vi "0037-Sub_measure4.vi"(6 "数値":dbl, 7 "温湿度データ":dbl[][](array[numeric]), 8 "error out":errorcluster, 11 "device":T1) -> (0 "error out 2":errorcluster caption="error out", 2 "出力配列":dbl[](array[numeric]), 3 "device 2":T1, 4 "配列":bool[](array[boolean]), 5 "温湿度データ 2":dbl[][](array[numeric]))   [LabVIEW 2014]
uses:
  <userlib>/LV-CP2112_2014/LVProject/private/CP2112_device.ctl
  <userlib>/LV-CP2112_2014/LVProject/private/CP2112_SMBUS_S0.ctl
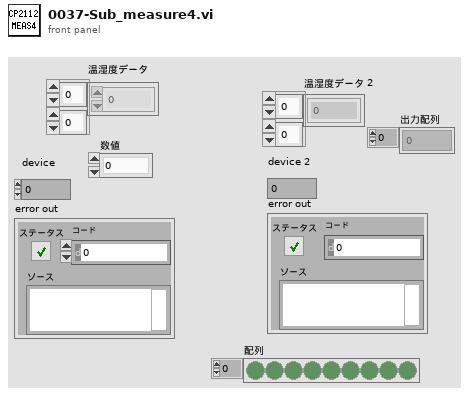
[diagram p1: front panel]
types:
  T1 = typedef "CP2112_device.ctl" = i32
  T2 = typedef "CP2112_SMBUS_S0.ctl" = enum8{"HID_SMBUS_S0_IDLE", "HID_SMBUS_S0_BUSY", "HID_SMBUS_S0_COMPLETE", "HID_SMBUS_S0_ERROR"}
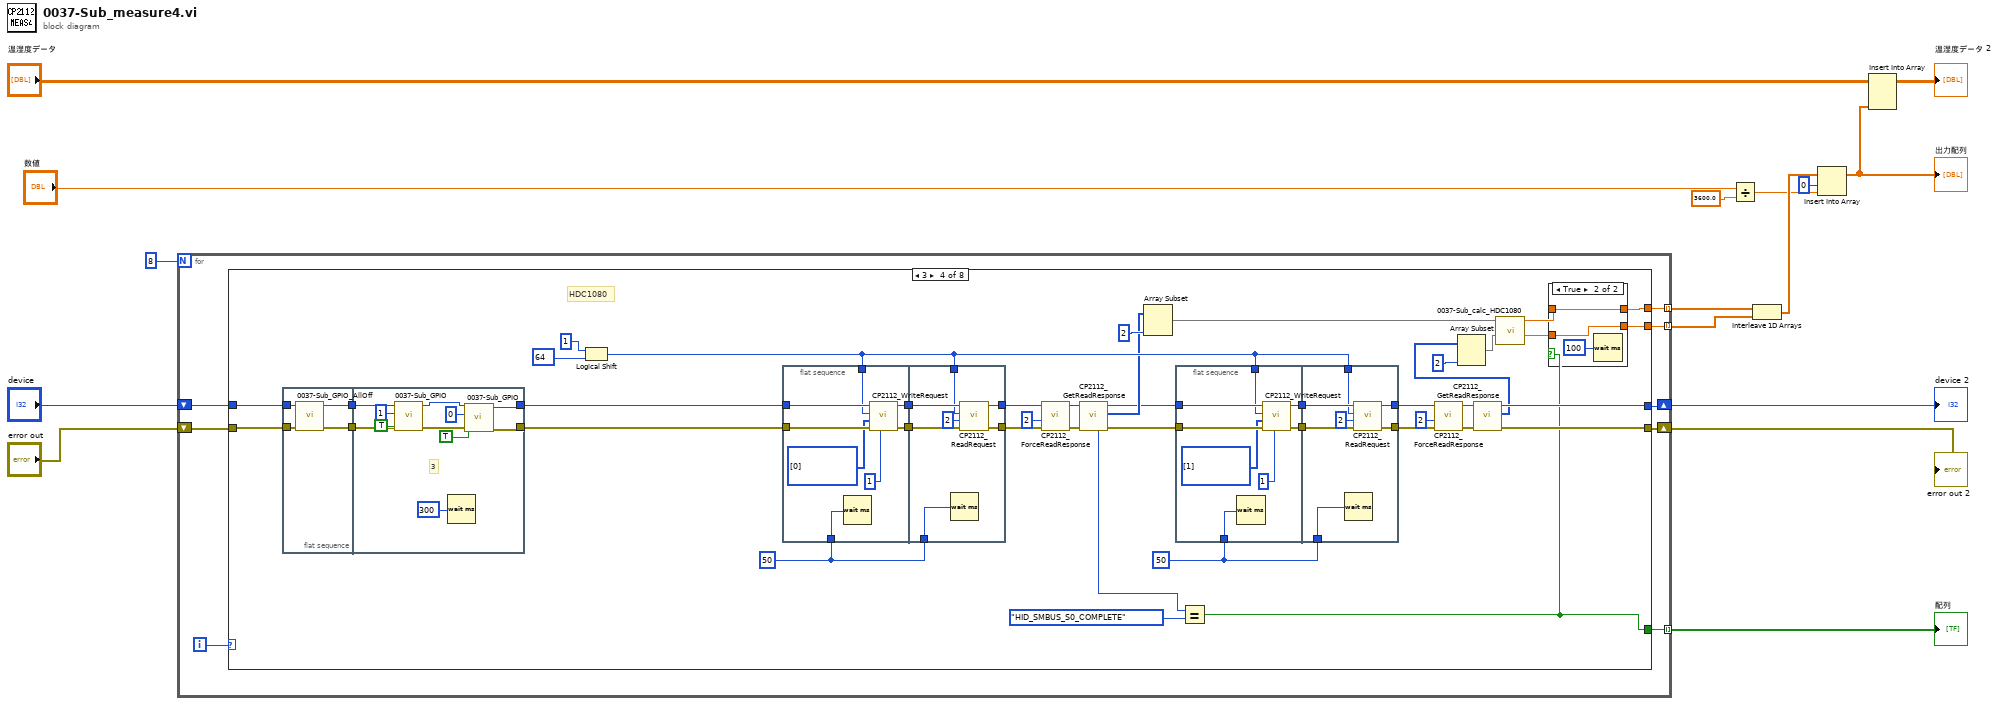
[diagram p0: block diagram]
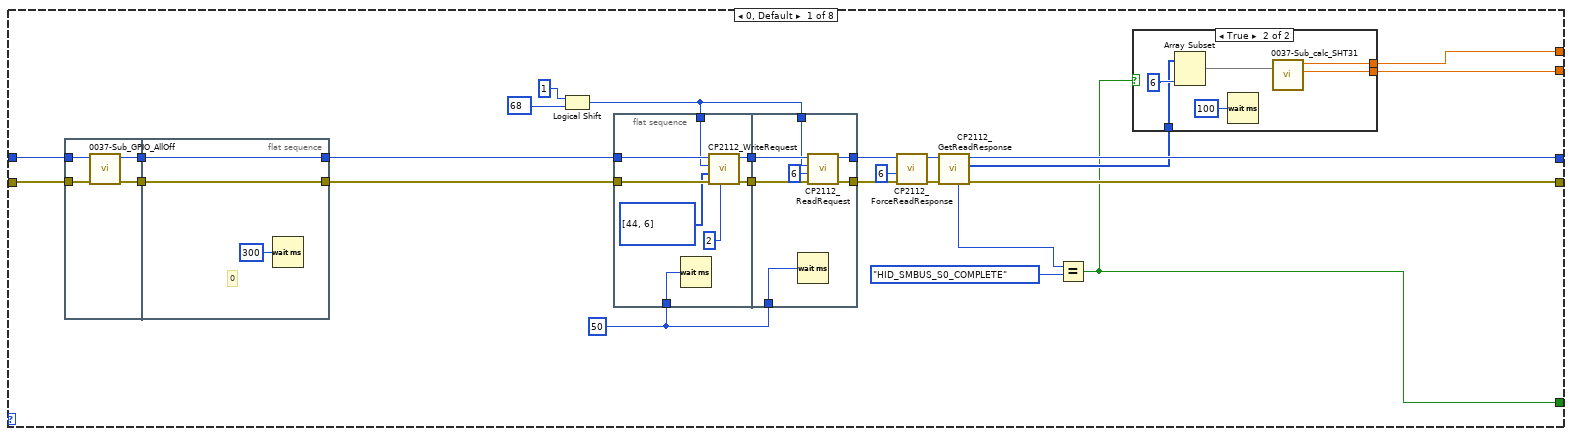
[diagram p2: hidden frame]
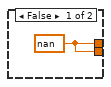
[diagram p3: hidden frame]
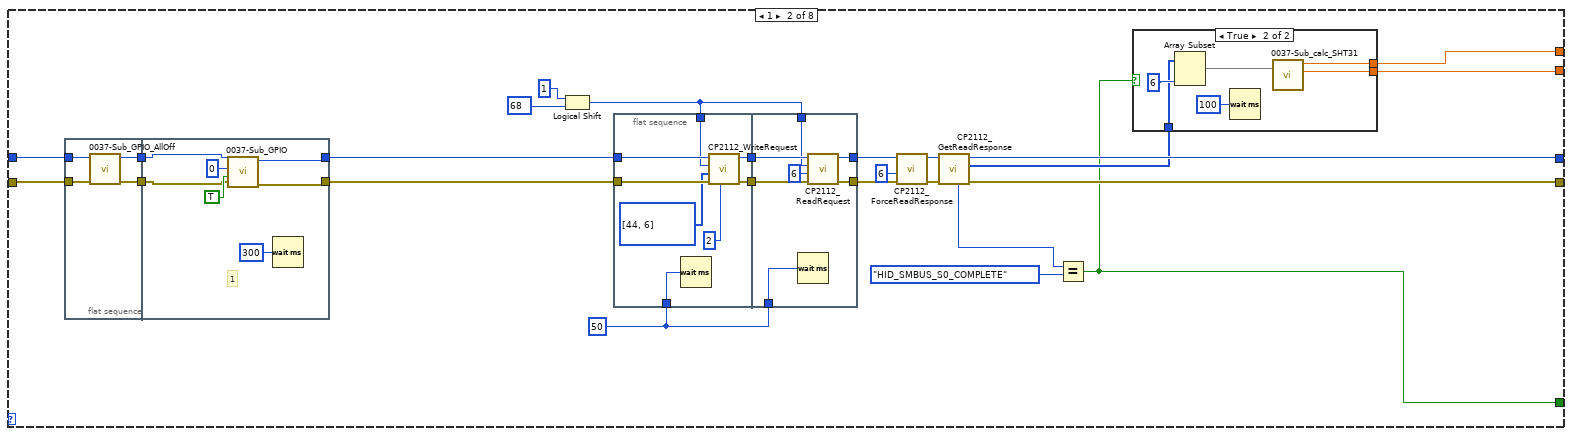
[diagram p4: hidden frame]
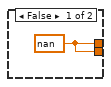
[diagram p5: hidden frame]
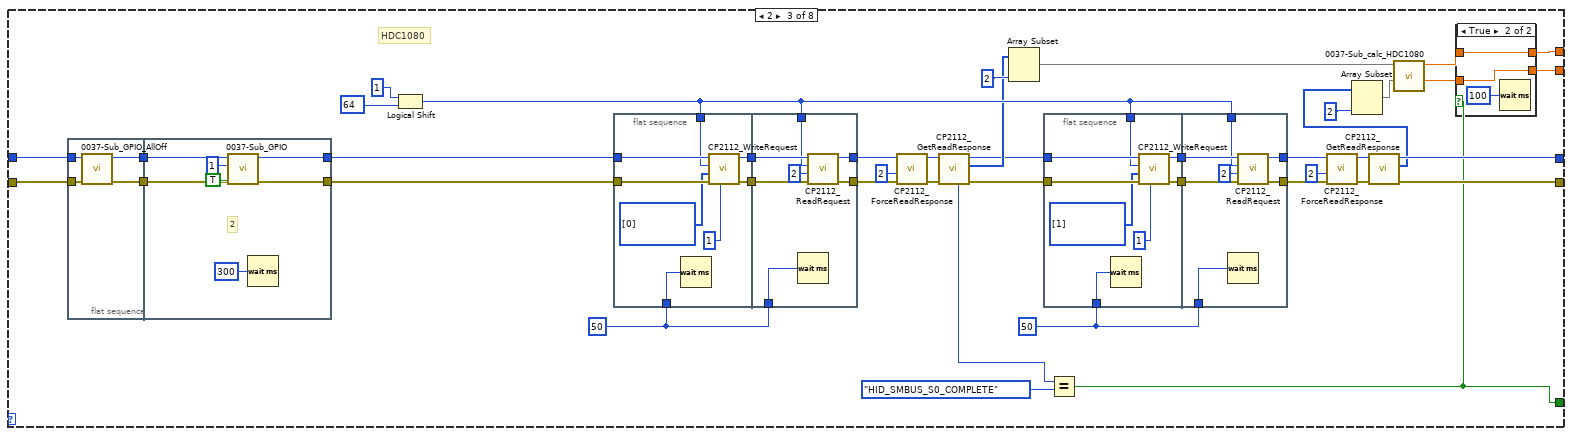
[diagram p6: hidden frame]
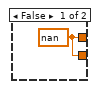
[diagram p7: hidden frame]
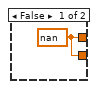
[diagram p8: hidden frame]
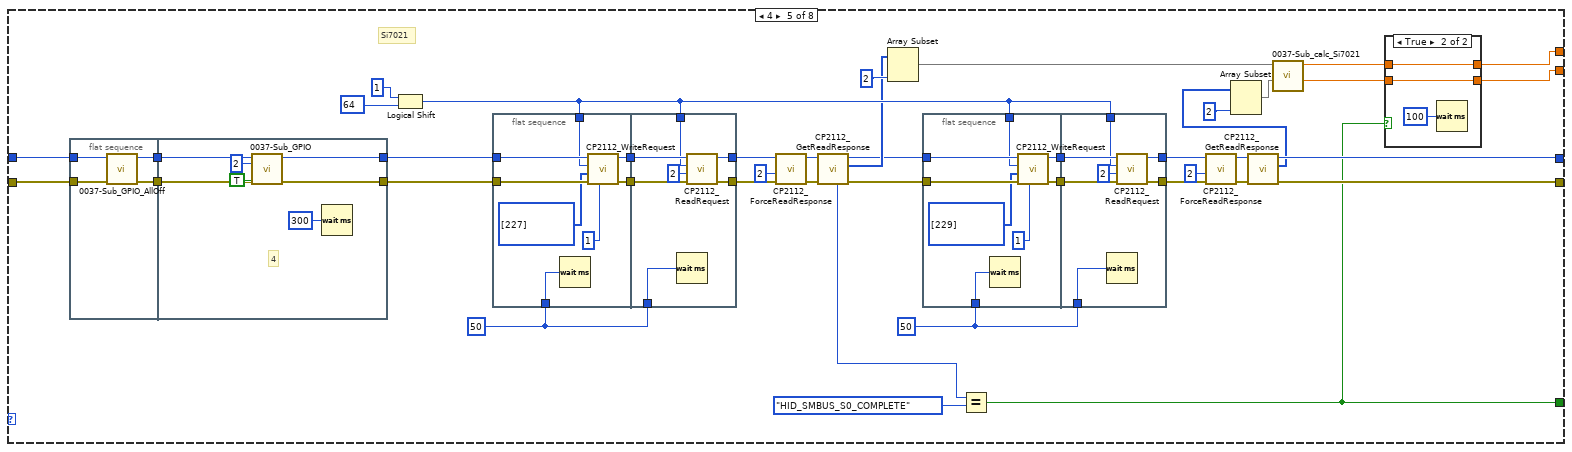
[diagram p9: hidden frame]
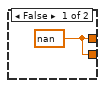
[diagram p10: hidden frame]
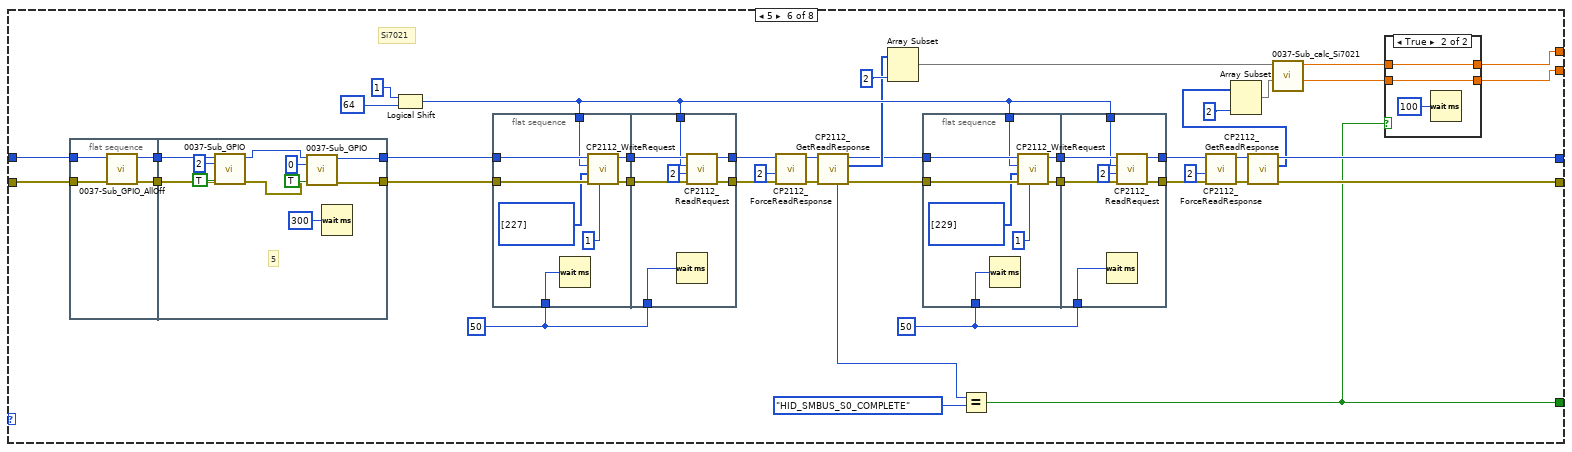
[diagram p11: hidden frame]
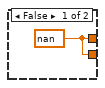
[diagram p12: hidden frame]
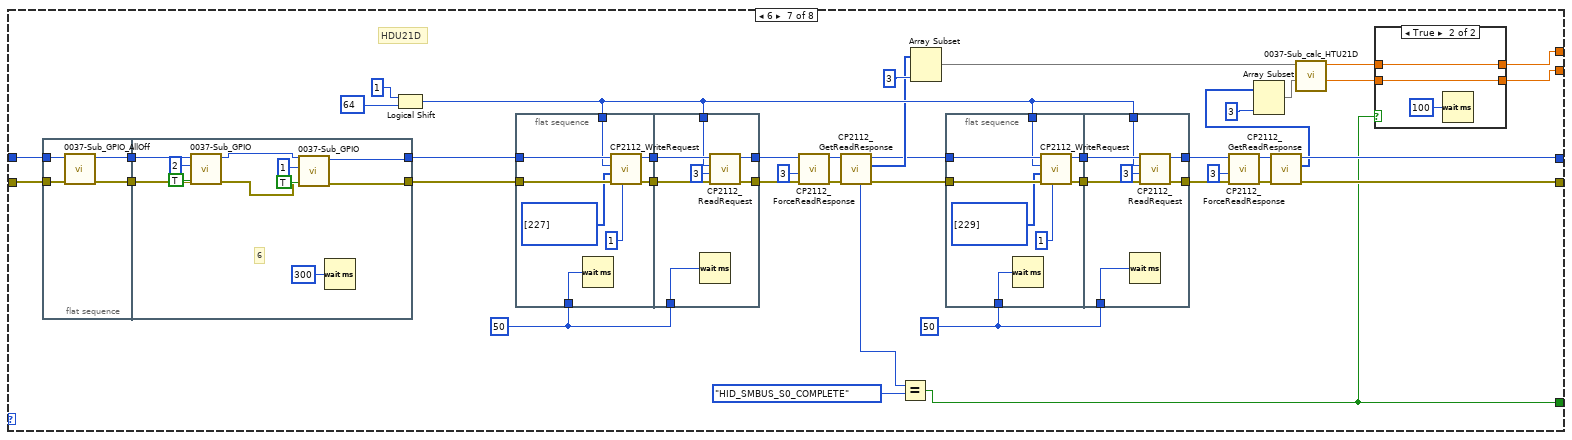
[diagram p13: hidden frame]
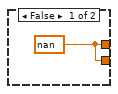
[diagram p14: hidden frame]
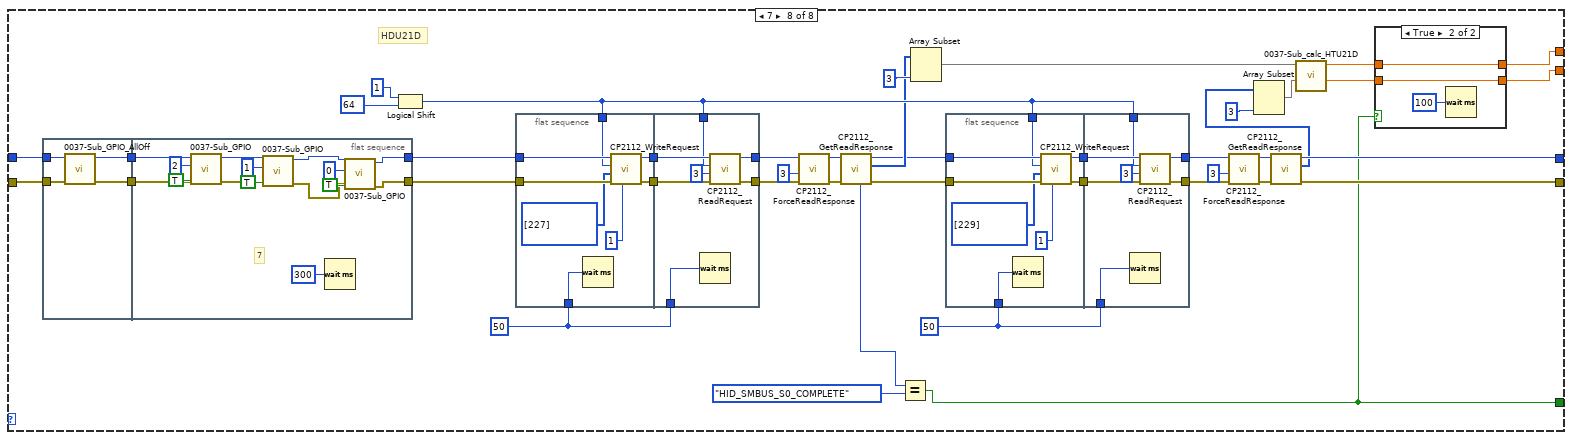
[diagram p15: hidden frame]
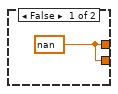
[diagram p16: hidden frame]
diagram:
  n1 = for {
    N: 8 -> [_]
    shift-right: [w22] -> w15
    shift-left: "error out" -> [w19]
    shift-right: [w23] -> w16
    shift-left: "device" -> [w18]
    tunnel: [w24] -> w14 mode=indexing
    tunnel: [w21] -> w9 mode=indexing
    tunnel: [w20] -> w8 mode=indexing
    i -> [w17]
    n2 = case shown="3" w17 {
      tunnel: [w25 w79 w137 w224 w319 w406 w497 w588] -> w24
      tunnel: [w41 w95 w172 w259 w350 w437 w528 w619] -> w23
      tunnel: [w42 w96 w173 w260 w351 w438 w529 w620] -> w22
      tunnel: [w44 w98 w139 w226 w318 w405 w496 w587] -> w21
      tunnel: [w43 w97 w141 w228 w316 w403 w494 w585] -> w20
      tunnel: w19 -> [w49 w103 w178 w265 w356 w443 w534 w625]
      tunnel: w18 -> [w48 w102 w177 w264 w355 w442 w533 w624]
      frame 0, Default {
        w30 = u32 50 ("ミリ秒待機時間")
        n3 = flat-sequence {
          tunnel: [w74] -> w40
          tunnel: [w72] -> w39
          tunnel: w48 -> [w75]
          tunnel: w49 -> [w73]
          tunnel: [w77] -> w27
          tunnel: [w78] -> w26
          tunnel: w40 -> [w77]
          tunnel: w39 -> [w78]
          frame #0 {
            n4 = call "0037-Sub_GPIO_AllOff.vi"("エラー出力 2"=w73, "device"=w75) -> ("エラー出力"=w72:errorcluster, "deviceOut"=w74:T1)  [unwired: 8 in]
          }
          frame #1 {
            # "0"
            n5 = Wait (ms)(milliseconds to wait=u32 300 ("ミリ秒待機時間")) -> ()  [unwired: 1 out]
          }
        }
        n6 = Logical Shift(y=1, x=68) -> (x << y=w45:i32)
        n7 = flat-sequence {
          tunnel: w26 -> [w64]
          tunnel: w27 -> [w63]
          tunnel: w45 -> [w58]
          tunnel: [w62] -> w38
          tunnel: [w61] -> w37
          tunnel: w30 -> [w57]
          tunnel: w38 -> [w69]
          tunnel: w37 -> [w68]
          tunnel: [w70] -> w32
          tunnel: [w67] -> w31
          tunnel: w45 -> [w66]
          tunnel: w30 -> [w65]
          frame #0 {
            n8 = Wait (ms)(milliseconds to wait=w57) -> ()  [unwired: 1 out]
            n9 = call <userlib>:"CP2112_WriteRequest.vi"("numBytesToWrite"=i16 2 ("numByteToRead"), "error in (no error)"=w64, "buffer"=u8[] [44, 6], "slaveAddress"=w58, "device"=w63) -> ("error out"=w62:errorcluster, "deviceOut"=w61:T1)  [unwired: 4 in, 1 out]
          }
          frame #1 {
            n10 = Wait (ms)(milliseconds to wait=w65) -> ()  [unwired: 1 out]
            n11 = call <userlib>:"CP2112_ReadRequest.vi"("error in (no error)"=w69, "numByteToRead"=i16 6, "slaveAddress"=w66, "device"=w68) -> ("error out"=w70:errorcluster, "deviceOut"=w67:T1)  [unwired: 5 in, 1 out]
          }
        }
        n12 = call <userlib>:"CP2112_ForceReadResponse.vi"("error in (no error)"=w32, "numByteToRead"=i16 6, "device"=w31) -> ("error out"=w36:errorcluster, "deviceOut"=w35:T1)  [unwired: 6 in, 1 out]
        n13 = call <userlib>:"CP2112_GetReadResponse.vi"("error in (no error)"=w36, "device"=w35) -> ("error out"=w42:errorcluster, "buffer"=w34:u8[], "deviceOut"=w41:T1, "HID_SMBUS_S0"=w29:T2)  [unwired: 4 in, 2 out]
        n14 = Equal?(x=w29, y=CP2112_SMBUS_S0."HID_SMBUS_S0_COMPLETE" ("HID_SMBUS_S0")) -> (x = y?=w25:bool)
        n15 = case shown="TRUE" w25 {
          tunnel: [w50 w56] -> w44
          tunnel: [w50 w55] -> w43
          tunnel: w34 -> [_ w52]
          frame False {
            w50 = nan ("数値 2")
          }
          frame True {
            n16 = Array Subset(array=w52, length=6 ("長さ")) -> (w54:u8[])  [unwired: 1 in]
            n17 = Wait (ms)(milliseconds to wait=u32 100 ("ミリ秒待機時間")) -> ()  [unwired: 1 out]
            n18 = call "0037-Sub_calc_SHT31.vi"("Data"=w54) -> ("数値"=w55:dbl, "数値 2"=w56:dbl)  [unwired: 9 in]
          }
        }
      }
      frame 1 {
        w84 = u32 50 ("ミリ秒待機時間")
        n19 = flat-sequence {
          tunnel: [w128] -> w94
          tunnel: [w126] -> w93
          tunnel: w102 -> [w129]
          tunnel: w103 -> [w127]
          tunnel: [w133] -> w81
          tunnel: [w132] -> w80
          tunnel: w94 -> [w130]
          tunnel: w93 -> [w131]
          frame #0 {
            n20 = call "0037-Sub_GPIO_AllOff.vi"("エラー出力 2"=w127, "device"=w129) -> ("エラー出力"=w126:errorcluster, "deviceOut"=w128:T1)  [unwired: 8 in]
          }
          frame #1 {
            # "1"
            n21 = call "0037-Sub_GPIO.vi"("エラー出力 2"=w131, "ブール"=TRUE, "GPIO"=u8 0, "device"=w130) -> ("エラー出力"=w132:errorcluster, "deviceOut"=w133:T1)  [unwired: 6 in]
            n22 = Wait (ms)(milliseconds to wait=u32 300 ("ミリ秒待機時間")) -> ()  [unwired: 1 out]
          }
        }
        n23 = Logical Shift(y=1, x=68) -> (x << y=w99:i32)
        n24 = flat-sequence {
          tunnel: w80 -> [w118]
          tunnel: w81 -> [w117]
          tunnel: w99 -> [w112]
          tunnel: [w116] -> w92
          tunnel: [w115] -> w91
          tunnel: w84 -> [w111]
          tunnel: w92 -> [w123]
          tunnel: w91 -> [w122]
          tunnel: [w124] -> w86
          tunnel: [w121] -> w85
          tunnel: w99 -> [w120]
          tunnel: w84 -> [w119]
          frame #0 {
            n25 = Wait (ms)(milliseconds to wait=w111) -> ()  [unwired: 1 out]
            n26 = call <userlib>:"CP2112_WriteRequest.vi"("numBytesToWrite"=i16 2 ("numByteToRead"), "error in (no error)"=w118, "buffer"=u8[] [44, 6], "slaveAddress"=w112, "device"=w117) -> ("error out"=w116:errorcluster, "deviceOut"=w115:T1)  [unwired: 4 in, 1 out]
          }
          frame #1 {
            n27 = Wait (ms)(milliseconds to wait=w119) -> ()  [unwired: 1 out]
            n28 = call <userlib>:"CP2112_ReadRequest.vi"("error in (no error)"=w123, "numByteToRead"=i16 6, "slaveAddress"=w120, "device"=w122) -> ("error out"=w124:errorcluster, "deviceOut"=w121:T1)  [unwired: 5 in, 1 out]
          }
        }
        n29 = call <userlib>:"CP2112_ForceReadResponse.vi"("error in (no error)"=w86, "numByteToRead"=i16 6, "device"=w85) -> ("error out"=w90:errorcluster, "deviceOut"=w89:T1)  [unwired: 6 in, 1 out]
        n30 = call <userlib>:"CP2112_GetReadResponse.vi"("error in (no error)"=w90, "device"=w89) -> ("error out"=w96:errorcluster, "buffer"=w88:u8[], "deviceOut"=w95:T1, "HID_SMBUS_S0"=w83:T2)  [unwired: 4 in, 2 out]
        n31 = Equal?(x=w83, y=CP2112_SMBUS_S0."HID_SMBUS_S0_COMPLETE" ("HID_SMBUS_S0")) -> (x = y?=w79:bool)
        n32 = case shown="TRUE" w79 {
          tunnel: [w104 w110] -> w98
          tunnel: [w104 w109] -> w97
          tunnel: w88 -> [_ w106]
          frame False {
            w104 = nan ("数値 2")
          }
          frame True {
            n33 = Array Subset(array=w106, length=6 ("長さ")) -> (w108:u8[])  [unwired: 1 in]
            n34 = Wait (ms)(milliseconds to wait=u32 100 ("ミリ秒待機時間")) -> ()  [unwired: 1 out]
            n35 = call "0037-Sub_calc_SHT31.vi"("Data"=w108) -> ("数値"=w109:dbl, "数値 2"=w110:dbl)  [unwired: 9 in]
          }
        }
      }
      frame 2 {
        w151 = u32 50 ("ミリ秒待機時間")
        w158 = u32 50 ("ミリ秒待機時間")
        # "HDC1080"
        n36 = flat-sequence {
          tunnel: [w215] -> w171
          tunnel: [w213] -> w170
          tunnel: w177 -> [w216]
          tunnel: w178 -> [w214]
          tunnel: [w223] -> w144
          tunnel: [w222] -> w145
          tunnel: w171 -> [w220]
          tunnel: w170 -> [w219]
          frame #0 {
            n37 = call "0037-Sub_GPIO_AllOff.vi"("エラー出力 2"=w214, "device"=w216) -> ("エラー出力"=w213:errorcluster, "deviceOut"=w215:T1)  [unwired: 8 in]
          }
          frame #1 {
            # "2"
            n38 = call "0037-Sub_GPIO.vi"("エラー出力 2"=w219, "ブール"=TRUE, "GPIO"=u8 1, "device"=w220) -> ("エラー出力"=w222:errorcluster, "deviceOut"=w223:T1)  [unwired: 6 in]
            n39 = Wait (ms)(milliseconds to wait=u32 300 ("ミリ秒待機時間")) -> ()  [unwired: 1 out]
          }
        }
        n40 = Logical Shift(y=1, x=64) -> (x << y=w174:i32)
        n41 = flat-sequence {
          tunnel: w145 -> [w205]
          tunnel: w144 -> [w204]
          tunnel: w174 -> [w199]
          tunnel: [w203] -> w169
          tunnel: [w202] -> w168
          tunnel: w158 -> [w198]
          tunnel: w169 -> [w210]
          tunnel: w168 -> [w209]
          tunnel: [w211] -> w160
          tunnel: [w208] -> w159
          tunnel: w174 -> [w207]
          tunnel: w158 -> [w206]
          frame #0 {
            n42 = Wait (ms)(milliseconds to wait=w198) -> ()  [unwired: 1 out]
            n43 = call <userlib>:"CP2112_WriteRequest.vi"("numBytesToWrite"=i16 1 ("numByteToRead"), "error in (no error)"=w205, "buffer"=u8[] [0], "slaveAddress"=w199, "device"=w204) -> ("error out"=w203:errorcluster, "deviceOut"=w202:T1)  [unwired: 4 in, 1 out]
          }
          frame #1 {
            n44 = Wait (ms)(milliseconds to wait=w206) -> ()  [unwired: 1 out]
            n45 = call <userlib>:"CP2112_ReadRequest.vi"("error in (no error)"=w210, "numByteToRead"=i16 2, "slaveAddress"=w207, "device"=w209) -> ("error out"=w211:errorcluster, "deviceOut"=w208:T1)  [unwired: 5 in, 1 out]
          }
        }
        n46 = call <userlib>:"CP2112_ForceReadResponse.vi"("error in (no error)"=w160, "numByteToRead"=i16 2, "device"=w159) -> ("error out"=w165:errorcluster, "deviceOut"=w164:T1)  [unwired: 6 in, 1 out]
        n47 = call <userlib>:"CP2112_GetReadResponse.vi"("error in (no error)"=w165, "device"=w164) -> ("error out"=w150:errorcluster, "buffer"=w162:u8[], "deviceOut"=w149:T1, "HID_SMBUS_S0"=w142:T2)  [unwired: 4 in, 2 out]
        n48 = Array Subset(array=w162, length=2 ("長さ")) -> (w157:u8[])  [unwired: 1 in]
        n49 = flat-sequence {
          tunnel: w150 -> [w190]
          tunnel: w149 -> [w189]
          tunnel: w174 -> [w184]
          tunnel: [w188] -> w167
          tunnel: [w187] -> w166
          tunnel: w151 -> [w183]
          tunnel: w167 -> [w195]
          tunnel: w166 -> [w194]
          tunnel: [w196] -> w153
          tunnel: [w193] -> w152
          tunnel: w174 -> [w192]
          tunnel: w151 -> [w191]
          frame #0 {
            n50 = Wait (ms)(milliseconds to wait=w183) -> ()  [unwired: 1 out]
            n51 = call <userlib>:"CP2112_WriteRequest.vi"("numBytesToWrite"=i16 1 ("numByteToRead"), "error in (no error)"=w190, "buffer"=u8[] [1], "slaveAddress"=w184, "device"=w189) -> ("error out"=w188:errorcluster, "deviceOut"=w187:T1)  [unwired: 4 in, 1 out]
          }
          frame #1 {
            n52 = Wait (ms)(milliseconds to wait=w191) -> ()  [unwired: 1 out]
            n53 = call <userlib>:"CP2112_ReadRequest.vi"("error in (no error)"=w195, "numByteToRead"=i16 2, "slaveAddress"=w192, "device"=w194) -> ("error out"=w196:errorcluster, "deviceOut"=w193:T1)  [unwired: 5 in, 1 out]
          }
        }
        n54 = Equal?(x=w142, y=CP2112_SMBUS_S0."HID_SMBUS_S0_COMPLETE" ("HID_SMBUS_S0")) -> (x = y?=w137:bool)
        n55 = call <userlib>:"CP2112_ForceReadResponse.vi"("error in (no error)"=w153, "numByteToRead"=i16 2, "device"=w152) -> ("error out"=w156:errorcluster, "deviceOut"=w155:T1)  [unwired: 6 in, 1 out]
        n56 = call <userlib>:"CP2112_GetReadResponse.vi"("error in (no error)"=w156, "device"=w155) -> ("error out"=w173:errorcluster, "buffer"=w146:u8[], "deviceOut"=w172:T1)  [unwired: 4 in, 3 out]
        n57 = Array Subset(array=w146, length=2 ("長さ")) -> (w147:u8[])  [unwired: 1 in]
        n58 = call "0037-Sub_calc_HDC1080.vi"("humi"=w147, "temp"=w157) -> ("humi"=w140:dbl, "temp"=w138:dbl)  [unwired: 7 in]
        n59 = case shown="TRUE" w137 {
          tunnel: [w179 w182] -> w141
          tunnel: w140 -> [_ w182]
          tunnel: [w179 w181] -> w139
          tunnel: w138 -> [_ w181]
          frame False {
            w179 = nan ("temp")
          }
          frame True {
            n60 = Wait (ms)(milliseconds to wait=u32 100 ("ミリ秒待機時間")) -> ()  [unwired: 1 out]
          }
        }
      }
      frame 3 {
        w238 = u32 50 ("ミリ秒待機時間")
        w245 = u32 50 ("ミリ秒待機時間")
        # "HDC1080"
        n61 = flat-sequence {
          tunnel: [w302] -> w258
          tunnel: [w300] -> w257
          tunnel: w264 -> [w303]
          tunnel: w265 -> [w301]
          tunnel: [w307] -> w231
          tunnel: [w306] -> w232
          tunnel: w258 -> [w313]
          tunnel: w257 -> [w312]
          frame #0 {
            n62 = call "0037-Sub_GPIO_AllOff.vi"("エラー出力 2"=w301, "device"=w303) -> ("エラー出力"=w300:errorcluster, "deviceOut"=w302:T1)  [unwired: 8 in]
          }
          frame #1 {
            # "3"
            n63 = call "0037-Sub_GPIO.vi"("エラー出力 2"=w312, "ブール"=TRUE, "GPIO"=u8 1, "device"=w313) -> ("エラー出力"=w305:errorcluster, "deviceOut"=w304:T1)  [unwired: 6 in]
            n64 = Wait (ms)(milliseconds to wait=u32 300 ("ミリ秒待機時間")) -> ()  [unwired: 1 out]
            n65 = call "0037-Sub_GPIO.vi"("エラー出力 2"=w305, "ブール"=TRUE, "GPIO"=u8 0, "device"=w304) -> ("エラー出力"=w306:errorcluster, "deviceOut"=w307:T1)  [unwired: 6 in]
          }
        }
        n66 = Logical Shift(y=1, x=64) -> (x << y=w261:i32)
        n67 = flat-sequence {
          tunnel: w232 -> [w292]
          tunnel: w231 -> [w291]
          tunnel: w261 -> [w286]
          tunnel: [w290] -> w256
          tunnel: [w289] -> w255
          tunnel: w245 -> [w285]
          tunnel: w256 -> [w297]
          tunnel: w255 -> [w296]
          tunnel: [w298] -> w247
          tunnel: [w295] -> w246
          tunnel: w261 -> [w294]
          tunnel: w245 -> [w293]
          frame #0 {
            n68 = Wait (ms)(milliseconds to wait=w285) -> ()  [unwired: 1 out]
            n69 = call <userlib>:"CP2112_WriteRequest.vi"("numBytesToWrite"=i16 1 ("numByteToRead"), "error in (no error)"=w292, "buffer"=u8[] [0], "slaveAddress"=w286, "device"=w291) -> ("error out"=w290:errorcluster, "deviceOut"=w289:T1)  [unwired: 4 in, 1 out]
          }
          frame #1 {
            n70 = Wait (ms)(milliseconds to wait=w293) -> ()  [unwired: 1 out]
            n71 = call <userlib>:"CP2112_ReadRequest.vi"("error in (no error)"=w297, "numByteToRead"=i16 2, "slaveAddress"=w294, "device"=w296) -> ("error out"=w298:errorcluster, "deviceOut"=w295:T1)  [unwired: 5 in, 1 out]
          }
        }
        n72 = call <userlib>:"CP2112_ForceReadResponse.vi"("error in (no error)"=w247, "numByteToRead"=i16 2, "device"=w246) -> ("error out"=w252:errorcluster, "deviceOut"=w251:T1)  [unwired: 6 in, 1 out]
        n73 = call <userlib>:"CP2112_GetReadResponse.vi"("error in (no error)"=w252, "device"=w251) -> ("error out"=w237:errorcluster, "buffer"=w249:u8[], "deviceOut"=w236:T1, "HID_SMBUS_S0"=w229:T2)  [unwired: 4 in, 2 out]
        n74 = Array Subset(array=w249, length=2 ("長さ")) -> (w244:u8[])  [unwired: 1 in]
        n75 = flat-sequence {
          tunnel: w237 -> [w277]
          tunnel: w236 -> [w276]
          tunnel: w261 -> [w271]
          tunnel: [w275] -> w254
          tunnel: [w274] -> w253
          tunnel: w238 -> [w270]
          tunnel: w254 -> [w282]
          tunnel: w253 -> [w281]
          tunnel: [w283] -> w240
          tunnel: [w280] -> w239
          tunnel: w261 -> [w279]
          tunnel: w238 -> [w278]
          frame #0 {
            n76 = Wait (ms)(milliseconds to wait=w270) -> ()  [unwired: 1 out]
            n77 = call <userlib>:"CP2112_WriteRequest.vi"("numBytesToWrite"=i16 1 ("numByteToRead"), "error in (no error)"=w277, "buffer"=u8[] [1], "slaveAddress"=w271, "device"=w276) -> ("error out"=w275:errorcluster, "deviceOut"=w274:T1)  [unwired: 4 in, 1 out]
          }
          frame #1 {
            n78 = Wait (ms)(milliseconds to wait=w278) -> ()  [unwired: 1 out]
            n79 = call <userlib>:"CP2112_ReadRequest.vi"("error in (no error)"=w282, "numByteToRead"=i16 2, "slaveAddress"=w279, "device"=w281) -> ("error out"=w283:errorcluster, "deviceOut"=w280:T1)  [unwired: 5 in, 1 out]
          }
        }
        n80 = Equal?(x=w229, y=CP2112_SMBUS_S0."HID_SMBUS_S0_COMPLETE" ("HID_SMBUS_S0")) -> (x = y?=w224:bool)
        n81 = call <userlib>:"CP2112_ForceReadResponse.vi"("error in (no error)"=w240, "numByteToRead"=i16 2, "device"=w239) -> ("error out"=w243:errorcluster, "deviceOut"=w242:T1)  [unwired: 6 in, 1 out]
        n82 = call <userlib>:"CP2112_GetReadResponse.vi"("error in (no error)"=w243, "device"=w242) -> ("error out"=w260:errorcluster, "buffer"=w233:u8[], "deviceOut"=w259:T1)  [unwired: 4 in, 3 out]
        n83 = Array Subset(array=w233, length=2 ("長さ")) -> (w234:u8[])  [unwired: 1 in]
        n84 = call "0037-Sub_calc_HDC1080.vi"("humi"=w234, "temp"=w244) -> ("humi"=w227:dbl, "temp"=w225:dbl)  [unwired: 7 in]
        n85 = case shown="TRUE" w224 {
          tunnel: [w266 w269] -> w228
          tunnel: w227 -> [_ w269]
          tunnel: [w266 w268] -> w226
          tunnel: w225 -> [_ w268]
          frame False {
            w266 = nan ("temp")
          }
          frame True {
            n86 = Wait (ms)(milliseconds to wait=u32 100 ("ミリ秒待機時間")) -> ()  [unwired: 1 out]
          }
        }
      }
      frame 4 {
        w329 = u32 50 ("ミリ秒待機時間")
        w336 = u32 50 ("ミリ秒待機時間")
        # "Si7021"
        n87 = flat-sequence {
          tunnel: [w393] -> w349
          tunnel: [w391] -> w348
          tunnel: w355 -> [w394]
          tunnel: w356 -> [w392]
          tunnel: [w401] -> w321
          tunnel: [w400] -> w322
          tunnel: w349 -> [w397]
          tunnel: w348 -> [w398]
          frame #0 {
            n88 = call "0037-Sub_GPIO_AllOff.vi"("エラー出力 2"=w392, "device"=w394) -> ("エラー出力"=w391:errorcluster, "deviceOut"=w393:T1)  [unwired: 8 in]
          }
          frame #1 {
            # "4"
            n89 = call "0037-Sub_GPIO.vi"("エラー出力 2"=w398, "ブール"=TRUE, "GPIO"=u8 2, "device"=w397) -> ("エラー出力"=w400:errorcluster, "deviceOut"=w401:T1)  [unwired: 6 in]
            n90 = Wait (ms)(milliseconds to wait=u32 300 ("ミリ秒待機時間")) -> ()  [unwired: 1 out]
          }
        }
        n91 = Logical Shift(y=1, x=64) -> (x << y=w352:i32)
        n92 = flat-sequence {
          tunnel: w322 -> [w383]
          tunnel: w321 -> [w382]
          tunnel: w352 -> [w377]
          tunnel: [w381] -> w347
          tunnel: [w380] -> w346
          tunnel: w336 -> [w376]
          tunnel: w347 -> [w388]
          tunnel: w346 -> [w387]
          tunnel: [w389] -> w338
          tunnel: [w386] -> w337
          tunnel: w352 -> [w385]
          tunnel: w336 -> [w384]
          frame #0 {
            n93 = Wait (ms)(milliseconds to wait=w376) -> ()  [unwired: 1 out]
            n94 = call <userlib>:"CP2112_WriteRequest.vi"("numBytesToWrite"=i16 1 ("numByteToRead"), "error in (no error)"=w383, "buffer"=u8[] [227], "slaveAddress"=w377, "device"=w382) -> ("error out"=w381:errorcluster, "deviceOut"=w380:T1)  [unwired: 4 in, 1 out]
          }
          frame #1 {
            n95 = Wait (ms)(milliseconds to wait=w384) -> ()  [unwired: 1 out]
            n96 = call <userlib>:"CP2112_ReadRequest.vi"("error in (no error)"=w388, "numByteToRead"=i16 2, "slaveAddress"=w385, "device"=w387) -> ("error out"=w389:errorcluster, "deviceOut"=w386:T1)  [unwired: 5 in, 1 out]
          }
        }
        n97 = call <userlib>:"CP2112_ForceReadResponse.vi"("error in (no error)"=w338, "numByteToRead"=i16 2, "device"=w337) -> ("error out"=w343:errorcluster, "deviceOut"=w342:T1)  [unwired: 6 in, 1 out]
        n98 = call <userlib>:"CP2112_GetReadResponse.vi"("error in (no error)"=w343, "device"=w342) -> ("error out"=w328:errorcluster, "buffer"=w340:u8[], "deviceOut"=w327:T1, "HID_SMBUS_S0"=w320:T2)  [unwired: 4 in, 2 out]
        n99 = Array Subset(array=w340, length=2 ("長さ")) -> (w335:u8[])  [unwired: 1 in]
        n100 = flat-sequence {
          tunnel: w328 -> [w368]
          tunnel: w327 -> [w367]
          tunnel: w352 -> [w362]
          tunnel: [w366] -> w345
          tunnel: [w365] -> w344
          tunnel: w329 -> [w361]
          tunnel: w345 -> [w373]
          tunnel: w344 -> [w372]
          tunnel: [w374] -> w331
          tunnel: [w371] -> w330
          tunnel: w352 -> [w370]
          tunnel: w329 -> [w369]
          frame #0 {
            n101 = Wait (ms)(milliseconds to wait=w361) -> ()  [unwired: 1 out]
            n102 = call <userlib>:"CP2112_WriteRequest.vi"("numBytesToWrite"=i16 1 ("numByteToRead"), "error in (no error)"=w368, "buffer"=u8[] [229], "slaveAddress"=w362, "device"=w367) -> ("error out"=w366:errorcluster, "deviceOut"=w365:T1)  [unwired: 4 in, 1 out]
          }
          frame #1 {
            n103 = Wait (ms)(milliseconds to wait=w369) -> ()  [unwired: 1 out]
            n104 = call <userlib>:"CP2112_ReadRequest.vi"("error in (no error)"=w373, "numByteToRead"=i16 2, "slaveAddress"=w370, "device"=w372) -> ("error out"=w374:errorcluster, "deviceOut"=w371:T1)  [unwired: 5 in, 1 out]
          }
        }
        n105 = Equal?(x=w320, y=CP2112_SMBUS_S0."HID_SMBUS_S0_COMPLETE" ("HID_SMBUS_S0")) -> (x = y?=w319:bool)
        n106 = call <userlib>:"CP2112_ForceReadResponse.vi"("error in (no error)"=w331, "numByteToRead"=i16 2, "device"=w330) -> ("error out"=w334:errorcluster, "deviceOut"=w333:T1)  [unwired: 6 in, 1 out]
        n107 = call <userlib>:"CP2112_GetReadResponse.vi"("error in (no error)"=w334, "device"=w333) -> ("error out"=w351:errorcluster, "buffer"=w324:u8[], "deviceOut"=w350:T1)  [unwired: 4 in, 3 out]
        n108 = Array Subset(array=w324, length=2 ("長さ")) -> (w325:u8[])  [unwired: 1 in]
        n109 = call "0037-Sub_calc_Si7021.vi"("humi"=w325, "temp"=w335) -> ("humi"=w315:dbl, "temp"=w317:dbl)  [unwired: 7 in]
        n110 = case shown="TRUE" w319 {
          tunnel: [w357 w360] -> w318
          tunnel: w317 -> [_ w360]
          tunnel: [w357 w359] -> w316
          tunnel: w315 -> [_ w359]
          frame False {
            w357 = nan ("temp")
          }
          frame True {
            n111 = Wait (ms)(milliseconds to wait=u32 100 ("ミリ秒待機時間")) -> ()  [unwired: 1 out]
          }
        }
      }
      frame 5 {
        w416 = u32 50 ("ミリ秒待機時間")
        w423 = u32 50 ("ミリ秒待機時間")
        # "Si7021"
        n112 = flat-sequence {
          tunnel: [w480] -> w436
          tunnel: [w478] -> w435
          tunnel: w442 -> [w481]
          tunnel: w443 -> [w479]
          tunnel: [w484] -> w408
          tunnel: [w485] -> w409
          tunnel: w436 -> [w490]
          tunnel: w435 -> [w491]
          frame #0 {
            n113 = call "0037-Sub_GPIO_AllOff.vi"("エラー出力 2"=w479, "device"=w481) -> ("エラー出力"=w478:errorcluster, "deviceOut"=w480:T1)  [unwired: 8 in]
          }
          frame #1 {
            # "5"
            n114 = call "0037-Sub_GPIO.vi"("エラー出力 2"=w491, "ブール"=TRUE, "GPIO"=u8 2, "device"=w490) -> ("エラー出力"=w483:errorcluster, "deviceOut"=w482:T1)  [unwired: 6 in]
            n115 = call "0037-Sub_GPIO.vi"("エラー出力 2"=w483, "ブール"=TRUE, "GPIO"=u8 0, "device"=w482) -> ("エラー出力"=w485:errorcluster, "deviceOut"=w484:T1)  [unwired: 6 in]
            n116 = Wait (ms)(milliseconds to wait=u32 300 ("ミリ秒待機時間")) -> ()  [unwired: 1 out]
          }
        }
        n117 = Logical Shift(y=1, x=64) -> (x << y=w439:i32)
        n118 = flat-sequence {
          tunnel: w409 -> [w470]
          tunnel: w408 -> [w469]
          tunnel: w439 -> [w464]
          tunnel: [w468] -> w434
          tunnel: [w467] -> w433
          tunnel: w423 -> [w463]
          tunnel: w434 -> [w475]
          tunnel: w433 -> [w474]
          tunnel: [w476] -> w425
          tunnel: [w473] -> w424
          tunnel: w439 -> [w472]
          tunnel: w423 -> [w471]
          frame #0 {
            n119 = Wait (ms)(milliseconds to wait=w463) -> ()  [unwired: 1 out]
            n120 = call <userlib>:"CP2112_WriteRequest.vi"("numBytesToWrite"=i16 1 ("numByteToRead"), "error in (no error)"=w470, "buffer"=u8[] [227], "slaveAddress"=w464, "device"=w469) -> ("error out"=w468:errorcluster, "deviceOut"=w467:T1)  [unwired: 4 in, 1 out]
          }
          frame #1 {
            n121 = Wait (ms)(milliseconds to wait=w471) -> ()  [unwired: 1 out]
            n122 = call <userlib>:"CP2112_ReadRequest.vi"("error in (no error)"=w475, "numByteToRead"=i16 2, "slaveAddress"=w472, "device"=w474) -> ("error out"=w476:errorcluster, "deviceOut"=w473:T1)  [unwired: 5 in, 1 out]
          }
        }
        n123 = call <userlib>:"CP2112_ForceReadResponse.vi"("error in (no error)"=w425, "numByteToRead"=i16 2, "device"=w424) -> ("error out"=w430:errorcluster, "deviceOut"=w429:T1)  [unwired: 6 in, 1 out]
        n124 = call <userlib>:"CP2112_GetReadResponse.vi"("error in (no error)"=w430, "device"=w429) -> ("error out"=w415:errorcluster, "buffer"=w427:u8[], "deviceOut"=w414:T1, "HID_SMBUS_S0"=w407:T2)  [unwired: 4 in, 2 out]
        n125 = Array Subset(array=w427, length=2 ("長さ")) -> (w422:u8[])  [unwired: 1 in]
        n126 = flat-sequence {
          tunnel: w415 -> [w455]
          tunnel: w414 -> [w454]
          tunnel: w439 -> [w449]
          tunnel: [w453] -> w432
          tunnel: [w452] -> w431
          tunnel: w416 -> [w448]
          tunnel: w432 -> [w460]
          tunnel: w431 -> [w459]
          tunnel: [w461] -> w418
          tunnel: [w458] -> w417
          tunnel: w439 -> [w457]
          tunnel: w416 -> [w456]
          frame #0 {
            n127 = Wait (ms)(milliseconds to wait=w448) -> ()  [unwired: 1 out]
            n128 = call <userlib>:"CP2112_WriteRequest.vi"("numBytesToWrite"=i16 1 ("numByteToRead"), "error in (no error)"=w455, "buffer"=u8[] [229], "slaveAddress"=w449, "device"=w454) -> ("error out"=w453:errorcluster, "deviceOut"=w452:T1)  [unwired: 4 in, 1 out]
          }
          frame #1 {
            n129 = Wait (ms)(milliseconds to wait=w456) -> ()  [unwired: 1 out]
            n130 = call <userlib>:"CP2112_ReadRequest.vi"("error in (no error)"=w460, "numByteToRead"=i16 2, "slaveAddress"=w457, "device"=w459) -> ("error out"=w461:errorcluster, "deviceOut"=w458:T1)  [unwired: 5 in, 1 out]
          }
        }
        n131 = Equal?(x=w407, y=CP2112_SMBUS_S0."HID_SMBUS_S0_COMPLETE" ("HID_SMBUS_S0")) -> (x = y?=w406:bool)
        n132 = call <userlib>:"CP2112_ForceReadResponse.vi"("error in (no error)"=w418, "numByteToRead"=i16 2, "device"=w417) -> ("error out"=w421:errorcluster, "deviceOut"=w420:T1)  [unwired: 6 in, 1 out]
        n133 = call <userlib>:"CP2112_GetReadResponse.vi"("error in (no error)"=w421, "device"=w420) -> ("error out"=w438:errorcluster, "buffer"=w411:u8[], "deviceOut"=w437:T1)  [unwired: 4 in, 3 out]
        n134 = Array Subset(array=w411, length=2 ("長さ")) -> (w412:u8[])  [unwired: 1 in]
        n135 = call "0037-Sub_calc_Si7021.vi"("humi"=w412, "temp"=w422) -> ("humi"=w402:dbl, "temp"=w404:dbl)  [unwired: 7 in]
        n136 = case shown="TRUE" w406 {
          tunnel: [w444 w447] -> w405
          tunnel: w404 -> [_ w447]
          tunnel: [w444 w446] -> w403
          tunnel: w402 -> [_ w446]
          frame False {
            w444 = nan ("temp")
          }
          frame True {
            n137 = Wait (ms)(milliseconds to wait=u32 100 ("ミリ秒待機時間")) -> ()  [unwired: 1 out]
          }
        }
      }
      frame 6 {
        w507 = u32 50 ("ミリ秒待機時間")
        w514 = u32 50 ("ミリ秒待機時間")
        # "HDU21D"
        n138 = flat-sequence {
          tunnel: [w571] -> w527
          tunnel: [w569] -> w526
          tunnel: w533 -> [w572]
          tunnel: w534 -> [w570]
          tunnel: [w577] -> w500
          tunnel: [w578] -> w501
          tunnel: w527 -> [w582]
          tunnel: w526 -> [w581]
          frame #0 {
            n139 = call "0037-Sub_GPIO_AllOff.vi"("エラー出力 2"=w570, "device"=w572) -> ("エラー出力"=w569:errorcluster, "deviceOut"=w571:T1)  [unwired: 8 in]
          }
          frame #1 {
            # "6"
            n140 = call "0037-Sub_GPIO.vi"("エラー出力 2"=w581, "ブール"=TRUE, "GPIO"=u8 2, "device"=w582) -> ("エラー出力"=w575:errorcluster, "deviceOut"=w576:T1)  [unwired: 6 in]
            n141 = call "0037-Sub_GPIO.vi"("エラー出力 2"=w575, "ブール"=TRUE, "GPIO"=u8 1, "device"=w576) -> ("エラー出力"=w578:errorcluster, "deviceOut"=w577:T1)  [unwired: 6 in]
            n142 = Wait (ms)(milliseconds to wait=u32 300 ("ミリ秒待機時間")) -> ()  [unwired: 1 out]
          }
        }
        n143 = Logical Shift(y=1, x=64) -> (x << y=w530:i32)
        n144 = flat-sequence {
          tunnel: w501 -> [w561]
          tunnel: w500 -> [w560]
          tunnel: w530 -> [w555]
          tunnel: [w559] -> w525
          tunnel: [w558] -> w524
          tunnel: w514 -> [w554]
          tunnel: w525 -> [w566]
          tunnel: w524 -> [w565]
          tunnel: [w567] -> w516
          tunnel: [w564] -> w515
          tunnel: w530 -> [w563]
          tunnel: w514 -> [w562]
          frame #0 {
            n145 = Wait (ms)(milliseconds to wait=w554) -> ()  [unwired: 1 out]
            n146 = call <userlib>:"CP2112_WriteRequest.vi"("numBytesToWrite"=i16 1 ("numByteToRead"), "error in (no error)"=w561, "buffer"=u8[] [227], "slaveAddress"=w555, "device"=w560) -> ("error out"=w559:errorcluster, "deviceOut"=w558:T1)  [unwired: 4 in, 1 out]
          }
          frame #1 {
            n147 = Wait (ms)(milliseconds to wait=w562) -> ()  [unwired: 1 out]
            n148 = call <userlib>:"CP2112_ReadRequest.vi"("error in (no error)"=w566, "numByteToRead"=i16 3, "slaveAddress"=w563, "device"=w565) -> ("error out"=w567:errorcluster, "deviceOut"=w564:T1)  [unwired: 5 in, 1 out]
          }
        }
        n149 = call <userlib>:"CP2112_ForceReadResponse.vi"("error in (no error)"=w516, "numByteToRead"=i16 3, "device"=w515) -> ("error out"=w521:errorcluster, "deviceOut"=w520:T1)  [unwired: 6 in, 1 out]
        n150 = call <userlib>:"CP2112_GetReadResponse.vi"("error in (no error)"=w521, "device"=w520) -> ("error out"=w506:errorcluster, "buffer"=w518:u8[], "deviceOut"=w505:T1, "HID_SMBUS_S0"=w498:T2)  [unwired: 4 in, 2 out]
        n151 = Equal?(x=w498, y=CP2112_SMBUS_S0."HID_SMBUS_S0_COMPLETE" ("HID_SMBUS_S0")) -> (x = y?=w497:bool)
        n152 = Array Subset(array=w518, length=3 ("長さ")) -> (w513:u8[])  [unwired: 1 in]
        n153 = flat-sequence {
          tunnel: w506 -> [w546]
          tunnel: w505 -> [w545]
          tunnel: w530 -> [w540]
          tunnel: [w544] -> w523
          tunnel: [w543] -> w522
          tunnel: w507 -> [w539]
          tunnel: w523 -> [w551]
          tunnel: w522 -> [w550]
          tunnel: [w552] -> w509
          tunnel: [w549] -> w508
          tunnel: w530 -> [w548]
          tunnel: w507 -> [w547]
          frame #0 {
            n154 = Wait (ms)(milliseconds to wait=w539) -> ()  [unwired: 1 out]
            n155 = call <userlib>:"CP2112_WriteRequest.vi"("numBytesToWrite"=i16 1 ("numByteToRead"), "error in (no error)"=w546, "buffer"=u8[] [229], "slaveAddress"=w540, "device"=w545) -> ("error out"=w544:errorcluster, "deviceOut"=w543:T1)  [unwired: 4 in, 1 out]
          }
          frame #1 {
            n156 = Wait (ms)(milliseconds to wait=w547) -> ()  [unwired: 1 out]
            n157 = call <userlib>:"CP2112_ReadRequest.vi"("error in (no error)"=w551, "numByteToRead"=i16 3, "slaveAddress"=w548, "device"=w550) -> ("error out"=w552:errorcluster, "deviceOut"=w549:T1)  [unwired: 5 in, 1 out]
          }
        }
        n158 = call <userlib>:"CP2112_ForceReadResponse.vi"("error in (no error)"=w509, "numByteToRead"=i16 3, "device"=w508) -> ("error out"=w512:errorcluster, "deviceOut"=w511:T1)  [unwired: 6 in, 1 out]
        n159 = call <userlib>:"CP2112_GetReadResponse.vi"("error in (no error)"=w512, "device"=w511) -> ("error out"=w529:errorcluster, "buffer"=w502:u8[], "deviceOut"=w528:T1)  [unwired: 4 in, 3 out]
        n160 = Array Subset(array=w502, length=3 ("長さ")) -> (w503:u8[])  [unwired: 1 in]
        n161 = call "0037-Sub_calc_HTU21D.vi"("humi"=w503, "temp"=w513) -> ("humi"=w493:dbl, "temp"=w495:dbl)  [unwired: 7 in]
        n162 = case shown="TRUE" w497 {
          tunnel: [w535 w538] -> w496
          tunnel: w495 -> [_ w538]
          tunnel: [w535 w537] -> w494
          tunnel: w493 -> [_ w537]
          frame False {
            w535 = nan ("temp")
          }
          frame True {
            n163 = Wait (ms)(milliseconds to wait=u32 100 ("ミリ秒待機時間")) -> ()  [unwired: 1 out]
          }
        }
      }
      frame 7 {
        w598 = u32 50 ("ミリ秒待機時間")
        w605 = u32 50 ("ミリ秒待機時間")
        # "HDU21D"
        n164 = flat-sequence {
          tunnel: [w662] -> w618
          tunnel: [w660] -> w617
          tunnel: w624 -> [w663]
          tunnel: w625 -> [w661]
          tunnel: [w666] -> w591
          tunnel: [w667] -> w592
          tunnel: w618 -> [w677]
          tunnel: w617 -> [w676]
          frame #0 {
            n165 = call "0037-Sub_GPIO_AllOff.vi"("エラー出力 2"=w661, "device"=w663) -> ("エラー出力"=w660:errorcluster, "deviceOut"=w662:T1)  [unwired: 8 in]
          }
          frame #1 {
            # "7"
            n166 = call "0037-Sub_GPIO.vi"("エラー出力 2"=w676, "ブール"=TRUE, "GPIO"=u8 2, "device"=w677) -> ("エラー出力"=w672:errorcluster, "deviceOut"=w673:T1)  [unwired: 6 in]
            n167 = call "0037-Sub_GPIO.vi"("エラー出力 2"=w672, "ブール"=TRUE, "GPIO"=u8 1, "device"=w673) -> ("エラー出力"=w664:errorcluster, "deviceOut"=w665:T1)  [unwired: 6 in]
            n168 = Wait (ms)(milliseconds to wait=u32 300 ("ミリ秒待機時間")) -> ()  [unwired: 1 out]
            n169 = call "0037-Sub_GPIO.vi"("エラー出力 2"=w664, "ブール"=TRUE, "GPIO"=u8 0, "device"=w665) -> ("エラー出力"=w667:errorcluster, "deviceOut"=w666:T1)  [unwired: 6 in]
          }
        }
        n170 = Logical Shift(y=1, x=64) -> (x << y=w621:i32)
        n171 = flat-sequence {
          tunnel: w592 -> [w652]
          tunnel: w591 -> [w651]
          tunnel: w621 -> [w646]
          tunnel: [w650] -> w616
          tunnel: [w649] -> w615
          tunnel: w605 -> [w645]
          tunnel: w616 -> [w657]
          tunnel: w615 -> [w656]
          tunnel: [w658] -> w607
          tunnel: [w655] -> w606
          tunnel: w621 -> [w654]
          tunnel: w605 -> [w653]
          frame #0 {
            n172 = Wait (ms)(milliseconds to wait=w645) -> ()  [unwired: 1 out]
            n173 = call <userlib>:"CP2112_WriteRequest.vi"("numBytesToWrite"=i16 1 ("numByteToRead"), "error in (no error)"=w652, "buffer"=u8[] [227], "slaveAddress"=w646, "device"=w651) -> ("error out"=w650:errorcluster, "deviceOut"=w649:T1)  [unwired: 4 in, 1 out]
          }
          frame #1 {
            n174 = Wait (ms)(milliseconds to wait=w653) -> ()  [unwired: 1 out]
            n175 = call <userlib>:"CP2112_ReadRequest.vi"("error in (no error)"=w657, "numByteToRead"=i16 3, "slaveAddress"=w654, "device"=w656) -> ("error out"=w658:errorcluster, "deviceOut"=w655:T1)  [unwired: 5 in, 1 out]
          }
        }
        n176 = call <userlib>:"CP2112_ForceReadResponse.vi"("error in (no error)"=w607, "numByteToRead"=i16 3, "device"=w606) -> ("error out"=w612:errorcluster, "deviceOut"=w611:T1)  [unwired: 6 in, 1 out]
        n177 = call <userlib>:"CP2112_GetReadResponse.vi"("error in (no error)"=w612, "device"=w611) -> ("error out"=w597:errorcluster, "buffer"=w609:u8[], "deviceOut"=w596:T1, "HID_SMBUS_S0"=w589:T2)  [unwired: 4 in, 2 out]
        n178 = Equal?(x=w589, y=CP2112_SMBUS_S0."HID_SMBUS_S0_COMPLETE" ("HID_SMBUS_S0")) -> (x = y?=w588:bool)
        n179 = Array Subset(array=w609, length=3 ("長さ")) -> (w604:u8[])  [unwired: 1 in]
        n180 = flat-sequence {
          tunnel: w597 -> [w637]
          tunnel: w596 -> [w636]
          tunnel: w621 -> [w631]
          tunnel: [w635] -> w614
          tunnel: [w634] -> w613
          tunnel: w598 -> [w630]
          tunnel: w614 -> [w642]
          tunnel: w613 -> [w641]
          tunnel: [w643] -> w600
          tunnel: [w640] -> w599
          tunnel: w621 -> [w639]
          tunnel: w598 -> [w638]
          frame #0 {
            n181 = Wait (ms)(milliseconds to wait=w630) -> ()  [unwired: 1 out]
            n182 = call <userlib>:"CP2112_WriteRequest.vi"("numBytesToWrite"=i16 1 ("numByteToRead"), "error in (no error)"=w637, "buffer"=u8[] [229], "slaveAddress"=w631, "device"=w636) -> ("error out"=w635:errorcluster, "deviceOut"=w634:T1)  [unwired: 4 in, 1 out]
          }
          frame #1 {
            n183 = Wait (ms)(milliseconds to wait=w638) -> ()  [unwired: 1 out]
            n184 = call <userlib>:"CP2112_ReadRequest.vi"("error in (no error)"=w642, "numByteToRead"=i16 3, "slaveAddress"=w639, "device"=w641) -> ("error out"=w643:errorcluster, "deviceOut"=w640:T1)  [unwired: 5 in, 1 out]
          }
        }
        n185 = call <userlib>:"CP2112_ForceReadResponse.vi"("error in (no error)"=w600, "numByteToRead"=i16 3, "device"=w599) -> ("error out"=w603:errorcluster, "deviceOut"=w602:T1)  [unwired: 6 in, 1 out]
        n186 = call <userlib>:"CP2112_GetReadResponse.vi"("error in (no error)"=w603, "device"=w602) -> ("error out"=w620:errorcluster, "buffer"=w593:u8[], "deviceOut"=w619:T1)  [unwired: 4 in, 3 out]
        n187 = Array Subset(array=w593, length=3 ("長さ")) -> (w594:u8[])  [unwired: 1 in]
        n188 = call "0037-Sub_calc_HTU21D.vi"("humi"=w594, "temp"=w604) -> ("humi"=w584:dbl, "temp"=w586:dbl)  [unwired: 7 in]
        n189 = case shown="TRUE" w588 {
          tunnel: [w626 w629] -> w587
          tunnel: w586 -> [_ w629]
          tunnel: [w626 w628] -> w585
          tunnel: w584 -> [_ w628]
          frame False {
            w626 = nan ("temp")
          }
          frame True {
            n190 = Wait (ms)(milliseconds to wait=u32 100 ("ミリ秒待機時間")) -> ()  [unwired: 1 out]
          }
        }
      }
    }
  }
  "配列" <- w14
  "device 2" <- w16
  "error out 2" <- w15
  n191 = Divide(x="数値", y=3600.0) -> (x/y=w4:dbl)
  n192 = Interleave 1D Arrays(w9, w8) -> (w7:dbl[])
  n193 = Insert Into Array(array=w7, index=0 ("指標"), new element=w4) -> (w2:dbl[])
  "出力配列" <- w2
  n194 = Insert Into Array(array="温湿度データ", new element=w2) -> (→"温湿度データ 2":dbl[][])  [unwired: 2 in]
